vi "Set_Power.vi"(8 "error in (no error)":errorcluster, 10 "Power":dbl, 11 "NKT in":refnum<class "NKT_Extreme.lvclass">) -> (0 "error out":errorcluster, 3 "NKT out":refnum<class "NKT_Extreme.lvclass">)   [LabVIEW 2020, in "NKT_Extreme.lvclass"]
doc: "Set overall power of Laser\nBe Carefull, Depending on Laser the expected value can be quite different\nAlways use Standard SI units!"
uses:
  <instrlib>/Classes/Laser/NKT/NKT_Extreme.lvclass
  <instrlib>/NKTP_API/NKTP_API.lvlib
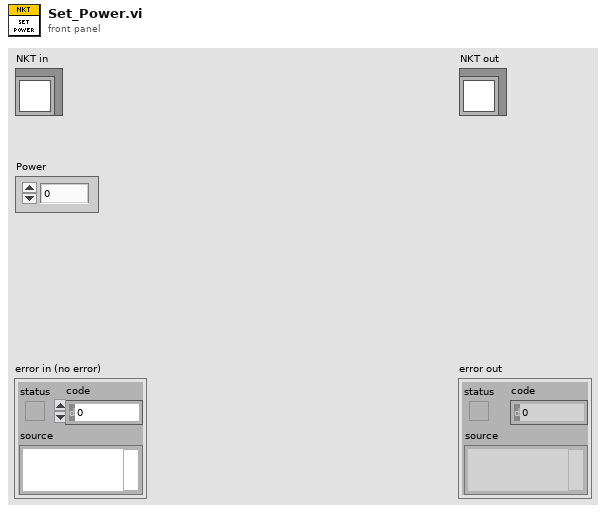
[diagram p1: front panel]
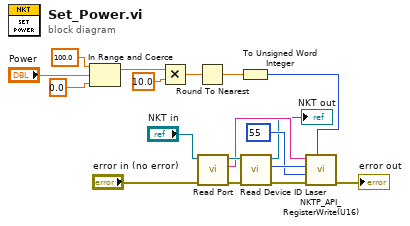
[diagram p0: block diagram]
diagram:
  n1 = In Range and Coerce(upper limit=100.0, x="Power", lower limit=0.0) -> (coerced(x)=w15:dbl)  [unwired: 1 out]
  n2 = Multiply(x=w15, y=10.0) -> (x*y=w13:dbl)
  n3 = Round To Nearest(number=w13) -> (nearest integer value=w12:dbl)
  n4 = call-dynamic "Read Port.vi"("error in (no error)"="error in (no error)", "NKT in"="NKT in") -> ("error out"=w7:errorcluster, "Port"=w6:string, "NKT out"=w8:refnum<class "NKT_Extreme.lvclass">)  [unwired: 7 in]
  n5 = To Unsigned Word Integer(number=w12) -> (unsigned 16bit integer=w11:u16)
  n6 = call-dynamic "Read Device ID Laser.vi"("error in (no error)"=w7, "NKT in"=w8) -> ("error out"=w3:errorcluster, "Device ID Laser"=w5:u8, "NKT out"=→"NKT out":refnum<class "NKT_Extreme.lvclass">)  [unwired: 7 in]
  n7 = call <instrlib>:"NKTP_API_RegisterWrite(U16).vi"("value"=w11, "error in"=w3, "regId"=u8 55, "devId"=w5, "portname"=w6) -> ("error out"=→"error out":errorcluster)  [unwired: 5 in, 1 out]
